vi "Testing VI.vi"() -> ()   [LabVIEW 2019]
panel:
  out "Boolean 5":bool
  out "String":string
  in  "Boolean 4":bool
  in  "Boolean 3":bool
  in  "Boolean":bool
  in  "Button":bool
  out "Boolean 2":bool
  in  "stop":bool
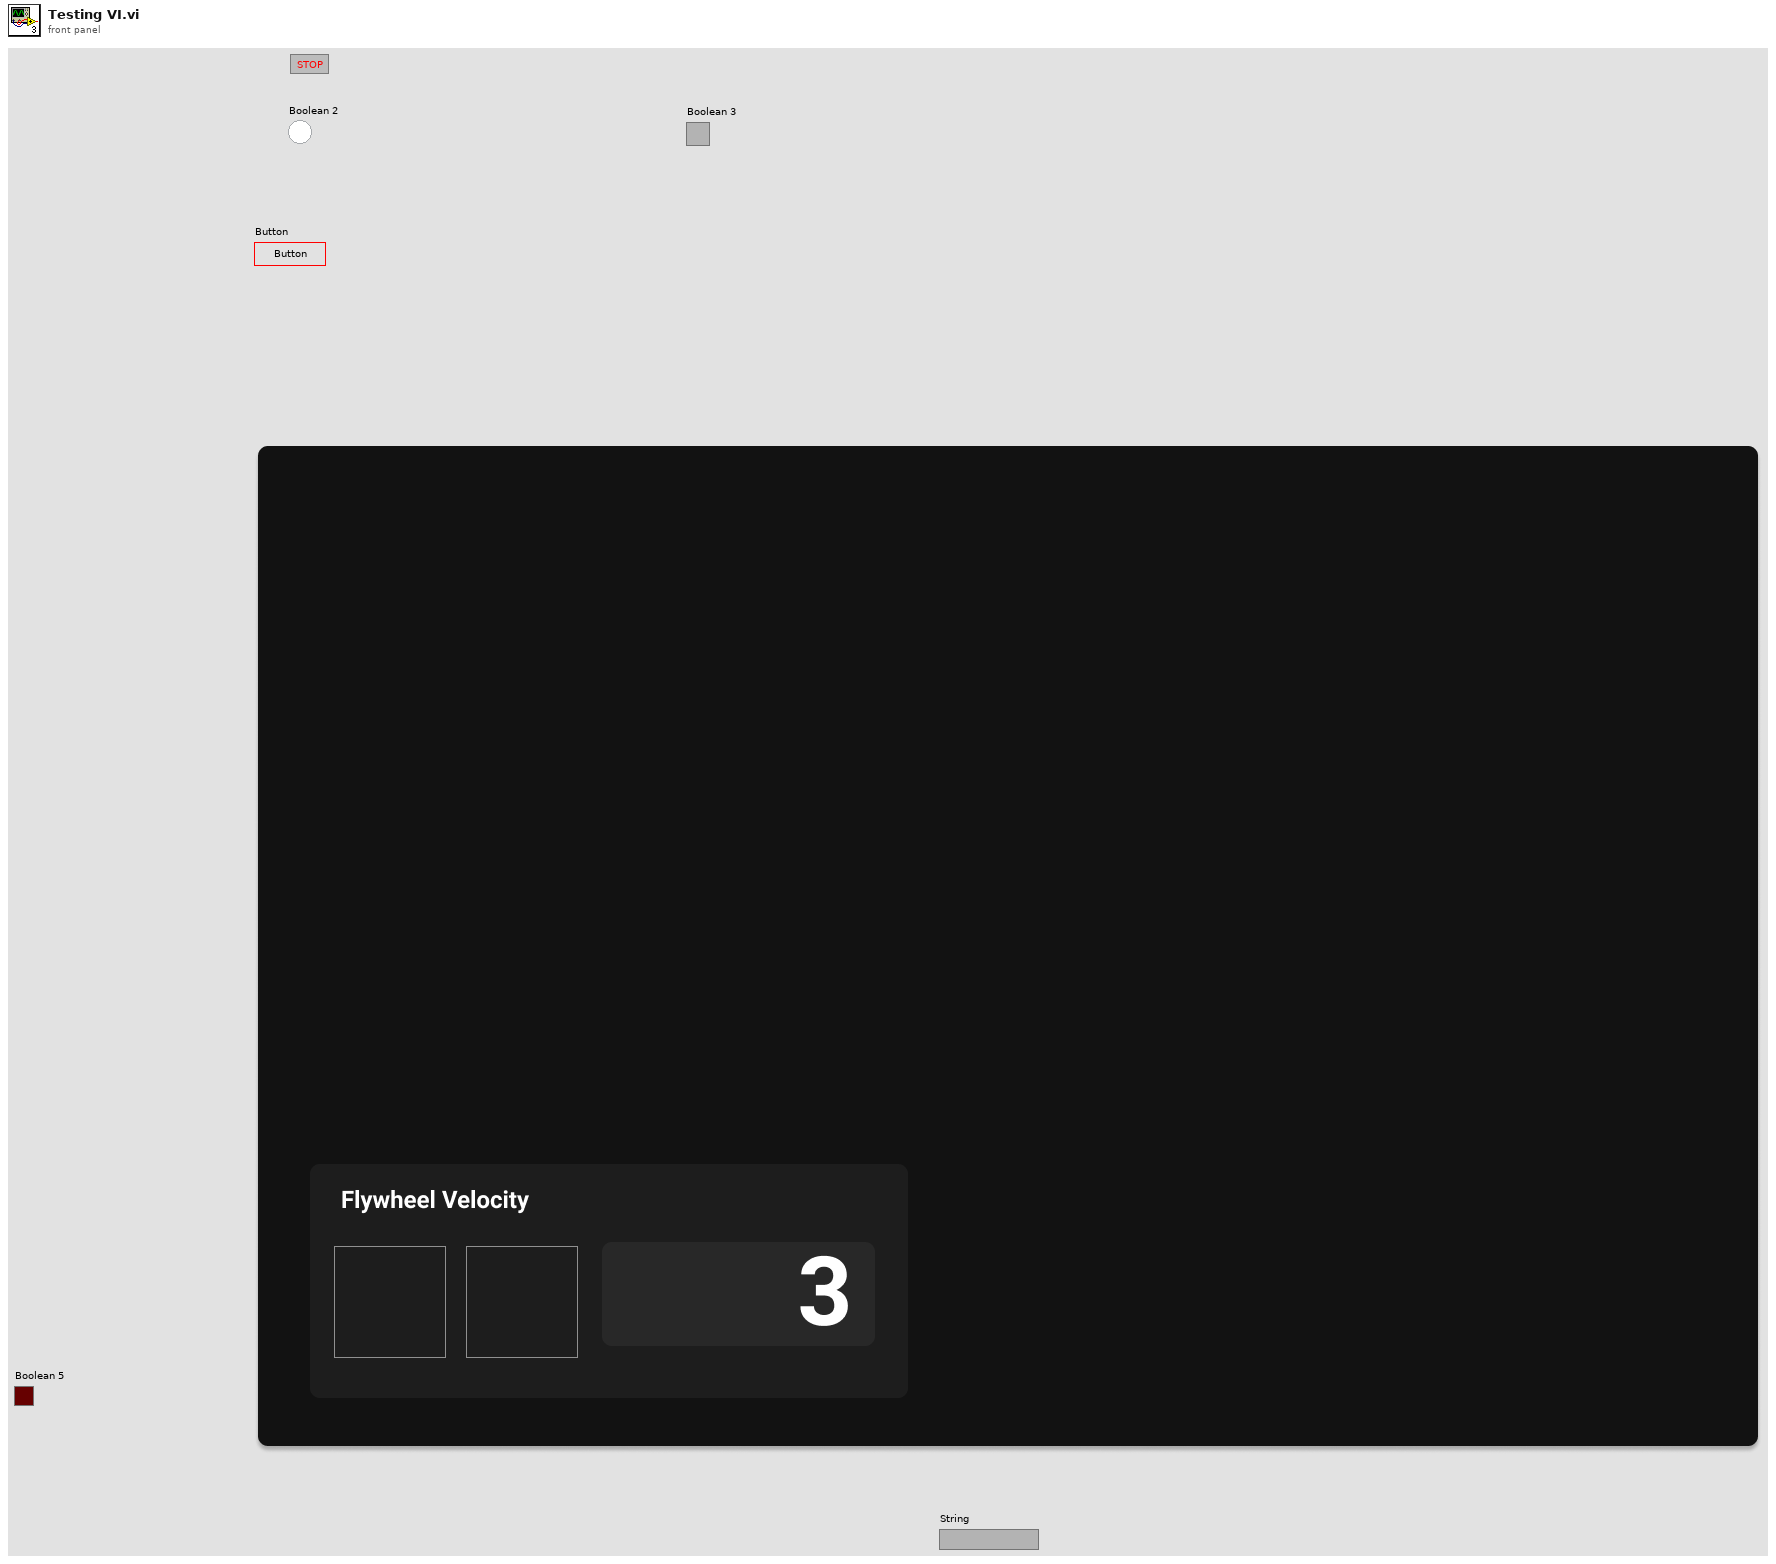
[diagram p1: front panel]
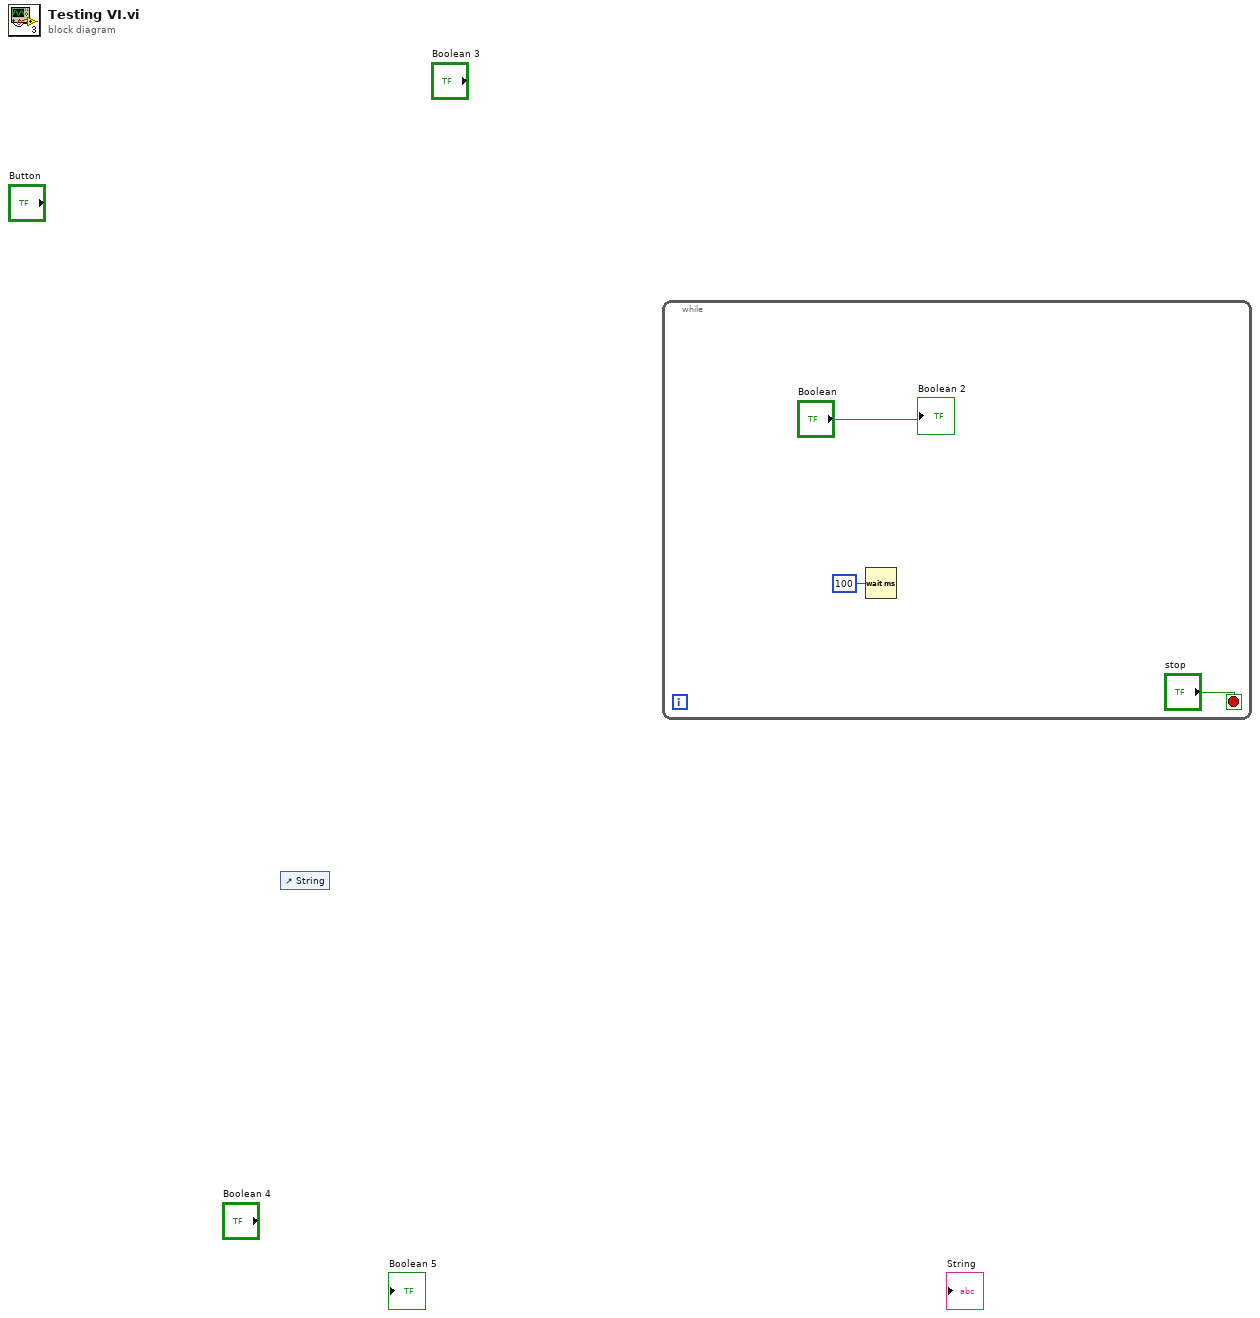
[diagram p0: block diagram]
diagram:
  n1 = control-ref of="String"() -> ()  [unwired: 1 out]
  n2 = while {
    stop <- "stop" stop-if-true
    n3 = Wait (ms)(milliseconds to wait=u32 100) -> ()  [unwired: 1 out]
    "Boolean 2" <- "Boolean"
  }
